vi "Str2BoolLua.vi"() -> ()   [LabVIEW 2013]
uses:
  TypeDefs/Active procedure variables.ctl
panel:
  out "(y value)":dbl
  out "x != 0?":bool
  out "error out":errorcluster
  in  "error in (no error)":errorcluster
  in  "Current Variable settings":T1[](array[typedef])
  in  "formula":string
  in  "Error Locator":string
  # "Our use of Lua:\n  - We are only working with doubles NOT bools\n  - Lua treats \"nil\" & \"false\" as false, anything else as true\n  - Therefore logical operators and, or, not will give\n       unexpected behavoir:\n  e.g.   1 and 0  will give 0 since \"and stops on false and \nreturns the last evaluated value\" (where 0 isn't 'nil' or 'false'!\n\nWe either need to add support to convert nil/false/true to\nappropriate DBL or we need to provide our own functions.\n\nimplement NOT: compare to 0 then use  a ? b : c (and b or c in lua):\n            DBL == 0 and 1 or 0  gives not(DBL)"
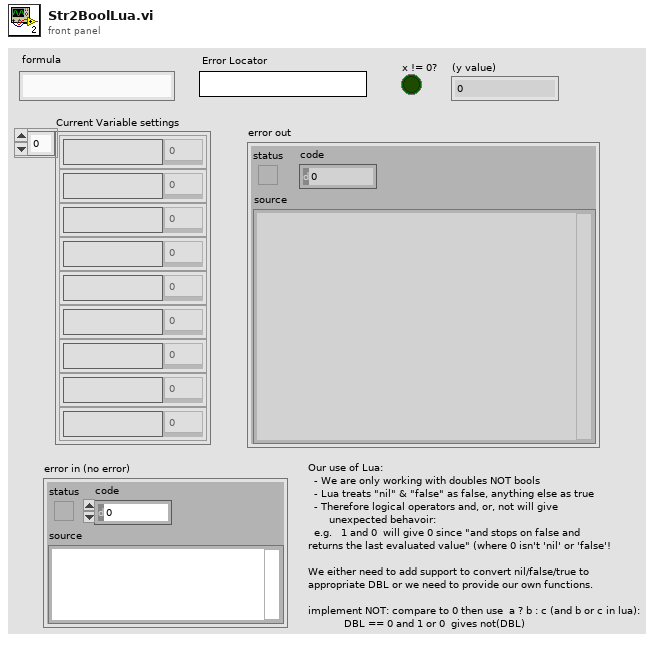
[diagram p1: front panel]
types:
  T1 = typedef "Active procedure variables.ctl" = cluster{"Procedure variable":string, "Value":dbl}
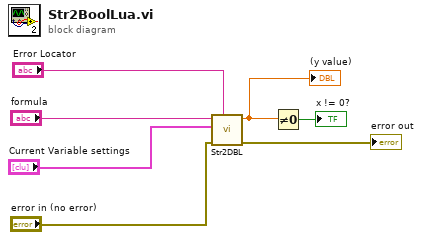
[diagram p0: block diagram]
diagram:
  n1 = call "Str2DBL.vi"("Error Locator"="Error Locator", "error in (no error)"="error in (no error)", "Current Variable settings"="Current Variable settings", "formula"="formula") -> ("error out"=→"error out":errorcluster, "y value"=w3:dbl)  [unwired: 4 in]
  "(y value)" <- w3
  n2 = Not Equal To 0?(x=w3) -> (x != 0?=→"x != 0?":bool)
